vi "Run Tests.vi"(8 "error in (no error)":errorcluster, 10 "Test Cases":refnum<class "Test Case.lvclass">[](array[class]), 11 "Test Executor in":refnum<class "Test Executor.lvclass">) -> (0 "error out":errorcluster, 2 "Test Results":refnum<class "Test Result.lvclass">[](array[class]), 3 "Test Executor out":refnum<class "Test Executor.lvclass">)   [LabVIEW 2017, in "Test Executor.lvclass"]
doc: "Runs the specified tests."
uses:
  Test Executor.lvclass
  Test Case/Test Case.lvclass
  Test Result/Test Result.lvclass
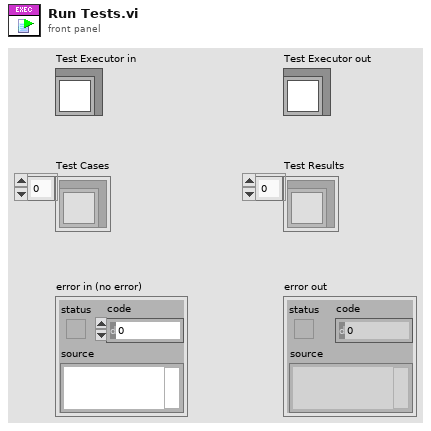
[diagram p1: front panel]
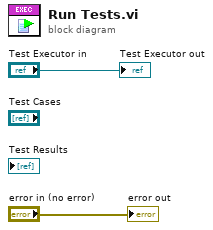
[diagram p0: block diagram]
diagram:
  "error out" <- "error in (no error)"
  "Test Executor out" <- "Test Executor in"
